vi "HWAsyncLoop.vi"(5 "HAL":refnum<queue>, 6 "Index":u32, 7 "HWAsync":refnum<queue>, 8 "error in":errorcluster, 10 "Async ACQ Notifier in":refnum<notifier>) -> (0 "error out":errorcluster)   [LabVIEW 2014, in "HWAsyncLoop.lvlib"]
uses:
  HWAsyncLoop.lvlib
  APIs/Message Queue/Message Cluster.ctl
  APIs/Data Queue/Async Acquisition Data Cluster.ctl
  DriverMasterAsync/builds/DriverMasterAsync.lvlibp/Modules/HAL/DriverMasterAsync/DriverMasterAsyncClass/DriverMasterAsync.lvclass
  Typedefs/HWAsync State.ctl
  <vilib>/Utility/error.llb/DialogType.ctl
  APIs/Message Queue/Enqueue Message (Single).vi
  <vilib>/Utility/LVLibp/NI_PackedLibraryUtility.lvlib
  APIs/Message Queue/WINFAS 2 Message Queue.lvlib
  APIs/Data Queue/WINFAS 2 Data Queue.lvlib
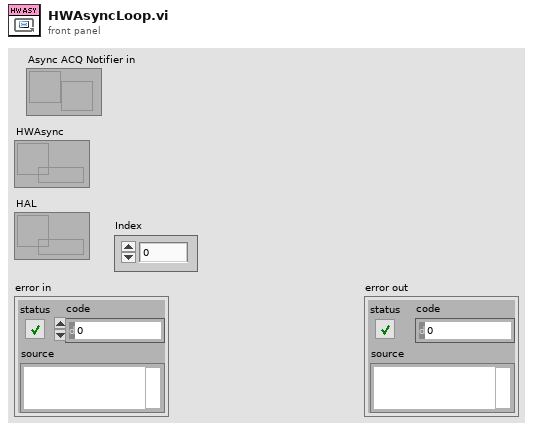
[diagram p1: front panel]
types:
  T1 = typedef "HWAsyncLoop.lvlib/HWAsync State.ctl" = enum16{"INIT", "Off", "Idle", "ACQ"}
  T2 = typedef "DialogType.ctl" = u16
  T3 = typedef "DriverMasterAsync.lvlibp/WINFAS 2 Data Queue.lvlib/Async Acquisition Data Cluster.ctl" = cluster{"Data":sgl[]}
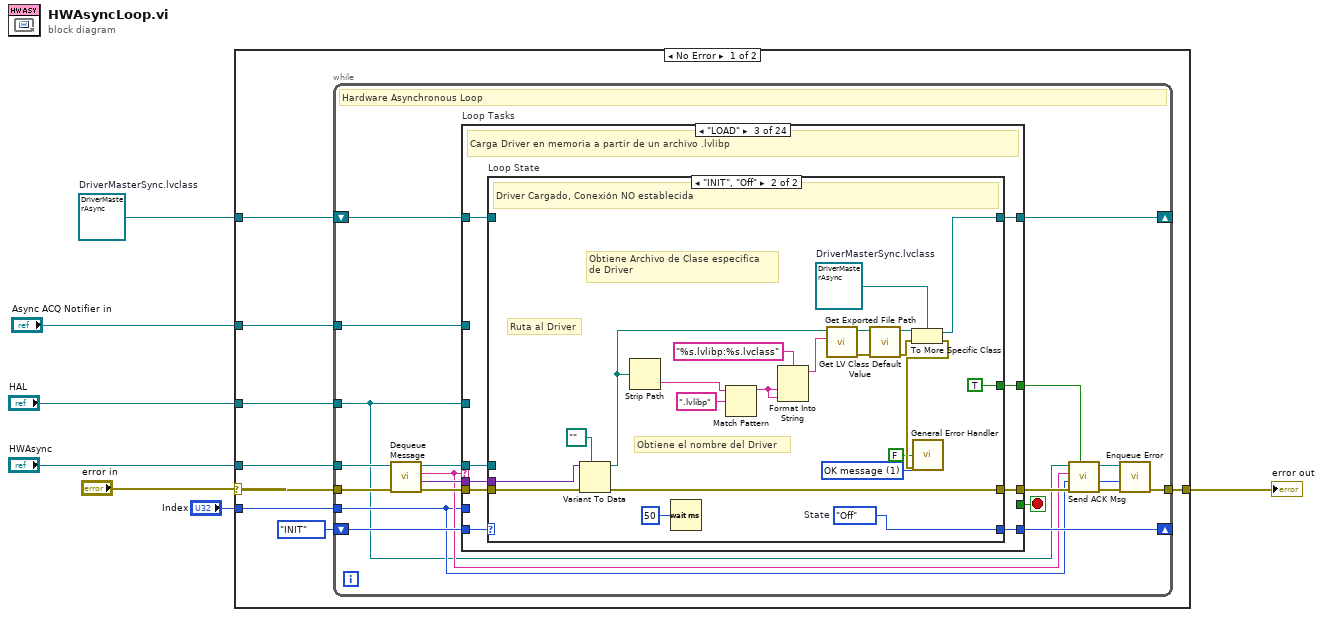
[diagram p0: block diagram]
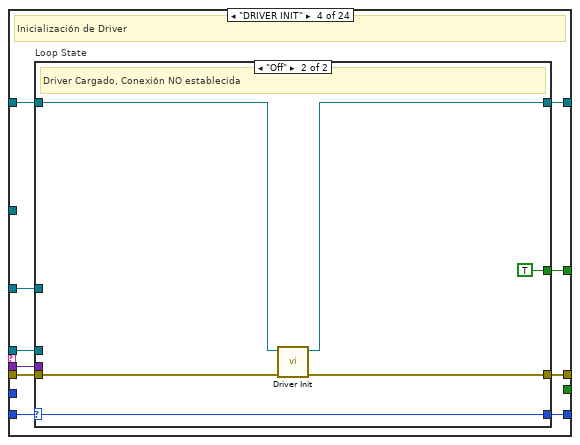
[diagram p5: hidden frame]
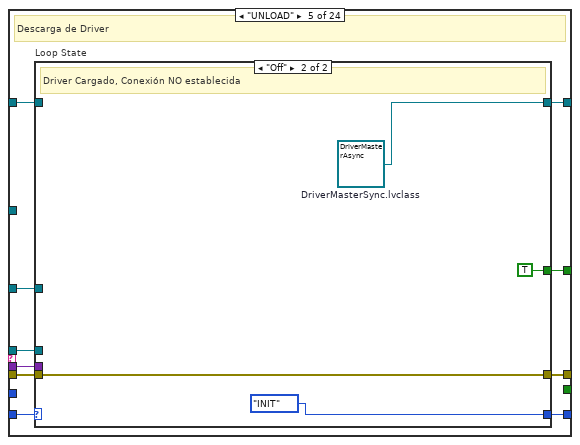
[diagram p7: hidden frame]
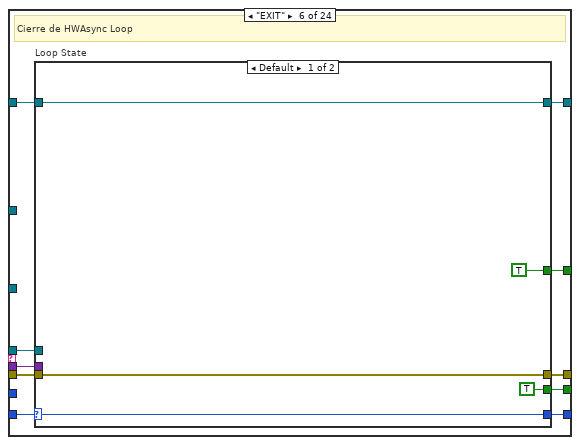
[diagram p9: hidden frame]
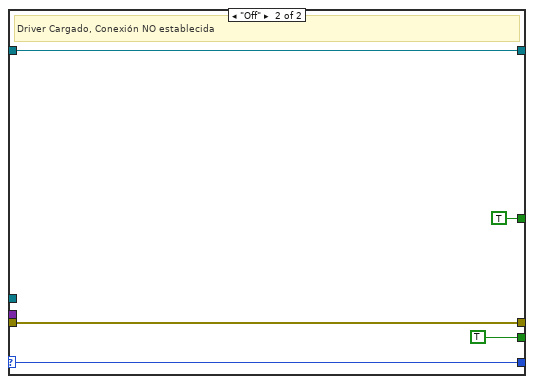
[diagram p10: hidden frame]
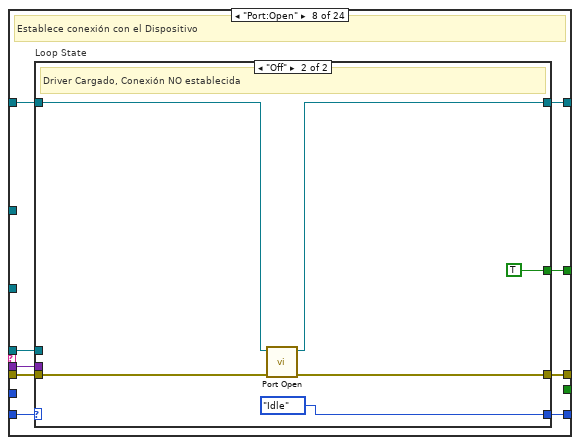
[diagram p12: hidden frame]
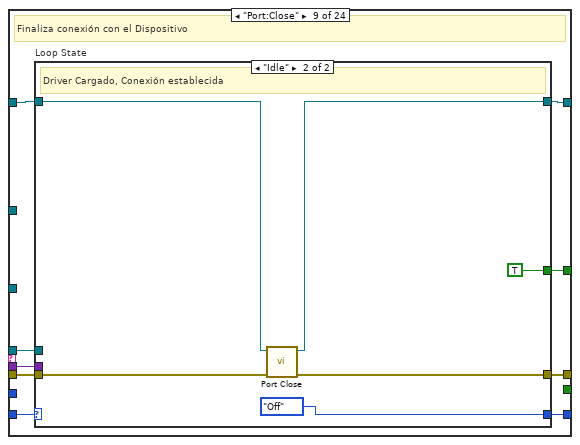
[diagram p14: hidden frame]
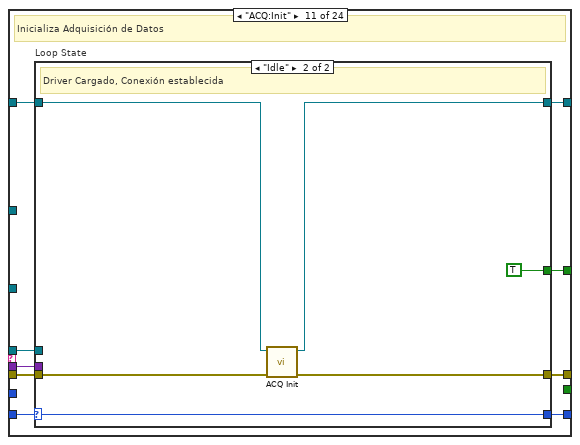
[diagram p17: hidden frame]
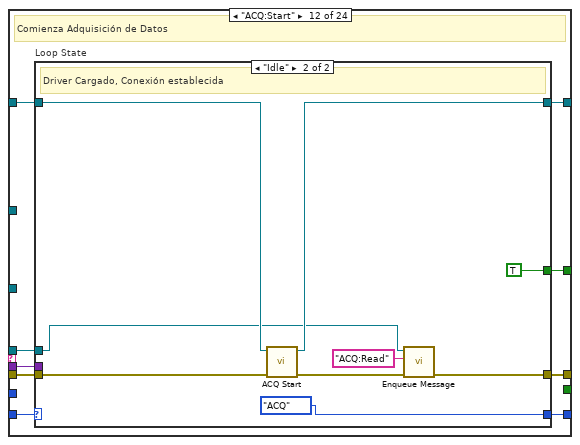
[diagram p19: hidden frame]
diagram:
  w3 = refnum<class "DriverMasterAsync.lvclass"> refnum  # DriverMasterSync.lvclass
  n1 = case shown="No Error" "error in" {
    selector: "error in" -> [w15 w435]
    tunnel: [w11 w435] -> w6
    tunnel: "HWAsync" -> [w14 _]
    tunnel: "HAL" -> [w12 _]
    tunnel: w3 -> [w10 _]
    tunnel: "Index" -> [w9 _]
    tunnel: "Async ACQ Notifier in" -> [w8 _]
    frame No Error {
      n2 = while {
        tunnel: w15 -> [w35]
        tunnel: w14 -> [w21]
        shift-right: [w30] -> _
        shift-left: HWAsync_State."INIT" ("State") -> [w29]
        tunnel: w12 -> [w17]
        tunnel: [w26] -> w11
        shift-right: [w32] -> _
        shift-left: w10 -> [w27]
        tunnel: w9 -> [w19]
        tunnel: w8 -> [w16]
        stop <- w34 stop-if-true
        # "Hardware Asynchronous Loop"
        n3 = call "Dequeue Message.vi"("error in (no error)"=w35, "Message Queue"=w21) -> ("error out"=w33:errorcluster, "Message Data"=w31:variant, "Message"=w20:string, "dup Message Queue"=w28:refnum<queue>)  [unwired: 6 in]
        n4 = case "Loop Tasks" shown="\"LOAD\"" w20 {
          tunnel: w28 -> [_ _ w46 w81 w100 w117 _ w139 w157 _ w178 w196 w219 w250 w269 _ w295 w313 w331 _ w353 w375 w396 w421]
          tunnel: w17 -> [_ _ _ w77 w96 _ _ _ _ _ _ _ w215 _ _ _ _ _ _ _ w349 w371 w392 w417]
          tunnel: [_ _ _ _ _ w113 _ _ _ _ _ _ _ _ _ _ _ _ _ _ _ _ _ _] -> w34
          tunnel: w33 -> [w38 w41 w49 w84 w103 w120 w134 w142 w160 w173 w181 w199 w222 w253 w272 w290 w298 w316 w334 w347 w356 w378 w399 w424]
          tunnel: [w38 w41 w47 w82 w101 w118 w134 w140 w158 w173 w179 w197 w220 w251 w270 w290 w296 w314 w332 w347 w354 w376 w397 w422] -> w22
          tunnel: w27 -> [w37 w40 w44 w79 w98 w115 w133 w137 w155 w172 w176 w194 w217 w248 w267 w289 w293 w311 w329 w346 w351 w373 w394 w419]
          tunnel: [w37 w40 w50 w85 w104 w121 w133 w143 w161 w172 w182 w200 w223 w254 w273 w289 w299 w317 w335 w346 w357 w379 w400 w425] -> w32
          tunnel: w31 -> [_ _ w48 w83 w102 w119 _ w141 w159 _ w180 w198 w221 w252 w271 _ w297 w315 w333 _ w355 w377 w398 w423]
          tunnel: [w36 w39 w43 w78 w97 w114 w132 w136 w154 w171 w175 w193 w216 w247 w266 w288 w292 w310 w328 w345 w350 w372 w393 w418] -> w30
          tunnel: w29 -> [w36 w39 w45 w80 w99 w116 w132 w138 w156 w171 w177 w195 w218 w249 w268 w288 w294 w312 w330 w345 w352 w374 w395 w420]
          tunnel: w19 -> [_ _ _ _ _ _ _ _ _ _ _ _ w214 _ _ _ _ _ _ _ _ _ w390 _]
          tunnel: [_ _ w42 w76 w95 w112 _ w135 w153 _ w174 w192 _ w246 w265 _ w291 w309 w327 _ w348 w370 w391 w416] -> w18
          tunnel: w16 -> [_ _ _ _ _ _ _ _ _ _ _ _ w213 _ w264 _ _ _ _ _ _ _ _ _]
          frame "----LOOP----" {
          }
          frame Default {
          }
          frame "LOAD" {
            # "Carga Driver en memoria a partir de un archivo .lvlibp"
            n5 = case "Loop State" shown="\"INIT\", \"Off\"" w45 {
              selector: w45 -> [w51 _]
              tunnel: [w53 w70] -> w50
              tunnel: w49 -> [w52 w69]
              tunnel: w48 -> [_ w68]
              tunnel: [w52 w59] -> w47
              tunnel: w46 -> [_ _]
              tunnel: w44 -> [w53 _]
              tunnel: [w51 w61] -> w43
              tunnel: [_ TRUE] -> w42
              frame Default {
              }
              frame "INIT", "Off" {
                w54 = T2 1 items=["no dialog", "OK message", "continue or stop message", "OK message + warnings", "continue/stop + warnings"] ("type of dialog (OK msg:1)")
                w61 = HWAsync_State."Off"  # State
                w71 = refnum<class "DriverMasterAsync.lvclass"> refnum  # DriverMasterSync.lvclass
                # "Ruta al Driver"
                # "Obtiene el nombre del Driver"
                # "Obtiene Archivo de Clase especifica\nde Driver"
                # "Driver Cargado, Conexión NO establecida"
                n6 = Variant To Data(error in=w69, type=path "", Variant=w68) -> (data=w64:path, error out=w59:errorcluster)
                n7 = Strip Path(path=w64) -> (name=w65:string)  [unwired: 1 out]
                n8 = Wait (ms)(milliseconds to wait=u32 50) -> ()  [unwired: 1 out]
                n9 = Match Pattern(string=w65, regular expression=".lvlibp") -> (before substring=w63:string)  [unwired: 1 in, 3 out]
                n10 = Format Into String(format string="%s.lvlibp:%s.lvclass", w63, w63) -> (resulting string=w74:string)  [unwired: 2 in, 1 out]
                n11 = call <vilib>:"Get Exported File Path.vi"("qualified name"=w74, "packed library path"=w64) -> ("error out"=w58:errorcluster, "path"=w75:path)  [unwired: 8 in]
                n12 = call <vilib>:"Get LV Class Default Value.vi"("error in (no error)"=w58, "class path"=w75) -> ("error out"=w57:errorcluster, "object"=w73:refnum<class>)  [unwired: 8 in]
                n13 = To More Specific Class(target class=w71, reference=w73, error in=w57) -> (specific class reference=w70:refnum<class "DriverMasterAsync.lvclass">, error out=w56:errorcluster)
                n14 = call <vilib>:"General Error Handler.vi"("search ni.com link visible?(T)"=FALSE, "type of dialog (OK msg:1)"=w54, "error in (no error)"=w56) -> ()  [unwired: 8 in, 5 out]
              }
            }
          }
          frame "DRIVER INIT" {
            # "Inicialización de Driver"
            n15 = case "Loop State" shown="\"Off\"" w80 {
              selector: w80 -> [w86 w94]
              tunnel: [w88 w91] -> w85
              tunnel: w84 -> [w87 w93]
              tunnel: w83 -> [_ _]
              tunnel: [w87 w89] -> w82
              tunnel: w81 -> [_ _]
              tunnel: w79 -> [w88 w92]
              tunnel: [w86 w94] -> w78
              tunnel: w77 -> [_ _]
              tunnel: [_ TRUE] -> w76
              frame Default {
              }
              frame "Off" {
                # "Driver Cargado, Conexión NO establecida"
                n16 = call-dynamic "Driver Init.vi"("error in (no error)"=w93, "DriverMasterAsync in"=w92) -> ("error out"=w89:errorcluster, "DriverMasterAsync out"=w91:refnum<class "DriverMasterAsync.lvclass">)  [unwired: 8 in]
              }
            }
          }
          frame "UNLOAD" {
            # "Descarga de Driver"
            n17 = case "Loop State" shown="\"Off\"" w99 {
              selector: w99 -> [w105 _]
              tunnel: [w107 w110] -> w104
              tunnel: w103 -> [w106 w109]
              tunnel: w102 -> [_ _]
              tunnel: [w106 w109] -> w101
              tunnel: w100 -> [_ _]
              tunnel: w98 -> [w107 _]
              tunnel: [w105 HWAsync_State."INIT" ("State")] -> w97
              tunnel: w96 -> [_ _]
              tunnel: [_ TRUE] -> w95
              frame Default {
              }
              frame "Off" {
                w110 = refnum<class "DriverMasterAsync.lvclass"> refnum  # DriverMasterSync.lvclass
                # "Driver Cargado, Conexión NO establecida"
              }
            }
          }
          frame "EXIT" {
            # "Cierre de HWAsync Loop"
            n18 = case "Loop State" shown="Default" w116 {
              selector: w116 -> [w124 w128]
              tunnel: [w126 w130] -> w121
              tunnel: w120 -> [w125 w129]
              tunnel: w119 -> [_ _]
              tunnel: [w125 w129] -> w118
              tunnel: w117 -> [_ _]
              tunnel: w115 -> [w126 w130]
              tunnel: [w124 w128] -> w114
              tunnel: [TRUE TRUE] -> w113
              tunnel: [TRUE TRUE] -> w112
              frame Default {
              }
              frame "Off" {
                # "Driver Cargado, Conexión NO establecida"
              }
            }
          }
          frame "----PORT----" {
          }
          frame "Port:Open" {
            # "Establece conexión con el Dispositivo"
            n19 = case "Loop State" shown="\"Off\"" w138 {
              selector: w138 -> [w144 _]
              tunnel: [w146 w149] -> w143
              tunnel: w142 -> [w145 w152]
              tunnel: w141 -> [_ _]
              tunnel: [w145 w151] -> w140
              tunnel: w139 -> [_ _]
              tunnel: w137 -> [w146 w150]
              tunnel: [w144 HWAsync_State."Idle" ("State")] -> w136
              tunnel: [_ TRUE] -> w135
              frame Default {
              }
              frame "Off" {
                # "Driver Cargado, Conexión NO establecida"
                n20 = call-dynamic "Port Open.vi"("error in (no error)"=w152, "DriverMasterAsync in"=w150) -> ("error out"=w151:errorcluster, "DriverMasterAsync out"=w149:refnum<class "DriverMasterAsync.lvclass">)  [unwired: 8 in]
              }
            }
          }
          frame "Port:Close" {
            # "Finaliza conexión con el Dispositivo"
            n21 = case "Loop State" shown="\"Idle\"" w156 {
              selector: w156 -> [w162 _]
              tunnel: [w164 w167] -> w161
              tunnel: w160 -> [w163 w170]
              tunnel: w159 -> [_ _]
              tunnel: [w163 w169] -> w158
              tunnel: w157 -> [_ _]
              tunnel: w155 -> [w164 w168]
              tunnel: [w162 HWAsync_State."Off" ("State")] -> w154
              tunnel: [_ TRUE] -> w153
              frame Default {
              }
              frame "Idle" {
                # "Driver Cargado, Conexión establecida"
                n22 = call-dynamic "Port Close.vi"("error in (no error)"=w170, "DriverMasterAsync in"=w168) -> ("error out"=w169:errorcluster, "DriverMasterAsync out"=w167:refnum<class "DriverMasterAsync.lvclass">)  [unwired: 8 in]
              }
            }
          }
          frame "----ACQ----" {
          }
          frame "ACQ:Init" {
            # "Inicializa Adquisición de Datos"
            n23 = case "Loop State" shown="\"Idle\"" w177 {
              selector: w177 -> [w183 w186]
              tunnel: [w185 w189] -> w182
              tunnel: w181 -> [w184 w191]
              tunnel: w180 -> [_ _]
              tunnel: [w184 w187] -> w179
              tunnel: w178 -> [_ _]
              tunnel: w176 -> [w185 w190]
              tunnel: [w183 w186] -> w175
              tunnel: [_ TRUE] -> w174
              frame Default {
              }
              frame "Idle" {
                # "Driver Cargado, Conexión establecida"
                n24 = call-dynamic "ACQ Init.vi"("error in (no error)"=w191, "DriverMasterAsync in"=w190) -> ("error out"=w187:errorcluster, "DriverMasterAsync out"=w189:refnum<class "DriverMasterAsync.lvclass">)  [unwired: 8 in]
              }
            }
          }
          frame "ACQ:Start" {
            # "Comienza Adquisición de Datos"
            n25 = case "Loop State" shown="\"Idle\"" w195 {
              selector: w195 -> [w201 _]
              tunnel: [w203 w210] -> w200
              tunnel: w199 -> [w202 w212]
              tunnel: w198 -> [_ _]
              tunnel: [w202 w206] -> w197
              tunnel: w196 -> [_ w205]
              tunnel: w194 -> [w203 w211]
              tunnel: [w201 HWAsync_State."ACQ" ("State")] -> w193
              tunnel: [_ TRUE] -> w192
              frame Default {
              }
              frame "Idle" {
                # "Driver Cargado, Conexión establecida"
                n26 = call-dynamic "ACQ Start.vi"("error in (no error)"=w212, "DriverMasterAsync in"=w211) -> ("error out"=w207:errorcluster, "DriverMasterAsync out"=w210:refnum<class "DriverMasterAsync.lvclass">)  [unwired: 8 in]
                n27 = call-poly "Enqueue Message.vi"("error in (no error)"=w207, "Message"="ACQ:Read", "Message Queue"=w205) -> ("error out"=w206:errorcluster)  [unwired: 7 in, 1 out]
              }
            }
          }
          frame "ACQ:Read" {
            # "Adquiere Datos"
            n28 = case "Loop State" shown="\"ACQ\"" w218 {
              selector: w218 -> [w224 w239]
              tunnel: [w226 w236] -> w223
              tunnel: w222 -> [w225 w241]
              tunnel: w221 -> [_ _]
              tunnel: [w225 w227] -> w220
              tunnel: w219 -> [_ w234]
              tunnel: w217 -> [w226 w240]
              tunnel: [w224 w239] -> w216
              tunnel: w215 -> [_ _]
              tunnel: w214 -> [_ _]
              tunnel: w213 -> [_ w230]
              frame Default {
              }
              frame "ACQ" {
                # "Adquiriendo Datos"
                n29 = for {
                  N: 100 -> [_]
                  tunnel: w240 -> [w244]
                  tunnel: [w243] -> w237
                  tunnel: w241 -> [w245]
                  tunnel: [w242] -> w238
                  stop <- w242 continue-if-true
                  n30 = call-dynamic "ACQ Read.vi"("error in (no error)"=w245, "DriverMasterAsync in"=w244) -> ("error out"=w242:errorcluster, "DriverMasterAsync out"=w243:refnum<class "DriverMasterAsync.lvclass">)  [unwired: 8 in]
                }
                n31 = call "Read ACQ Data.vi"("error in (no error)"=w238, "DriverMasterAsync in"=w237) -> ("error out"=w232:errorcluster, "ACQ Data"=w231:T3, "DriverMasterAsync out"=w236:refnum<class "DriverMasterAsync.lvclass">)  [unwired: 7 in]
                n32 = call "Send Async ACQ Notification.vi"("error in (no error)"=w232, "Async ACQ"=w231, "Async ACQ Notifier in"=w230) -> ("error out"=w229:errorcluster)  [unwired: 7 in, 1 out]
                n33 = call-poly "Enqueue Message.vi"("error in (no error)"=w232, "Message"="ACQ:Read", "Message Queue"=w234) -> ("error out"=w228:errorcluster)  [unwired: 7 in, 1 out]
                n34 = Merge Errors(w229, w228) -> (w227:errorcluster)
              }
            }
          }
          frame "ACQ:Stop" {
            # "Detiene Adquisición de Datos"
            n35 = case "Loop State" shown="\"ACQ\"" w249 {
              selector: w249 -> [w255 _]
              tunnel: [w257 w260] -> w254
              tunnel: w253 -> [w256 w263]
              tunnel: w252 -> [_ _]
              tunnel: [w256 w262] -> w251
              tunnel: w250 -> [_ _]
              tunnel: w248 -> [w257 w261]
              tunnel: [w255 HWAsync_State."Idle" ("State")] -> w247
              tunnel: [_ TRUE] -> w246
              frame Default {
              }
              frame "ACQ" {
                # "Adquiriendo Datos"
                n36 = call-dynamic "ACQ Stop.vi"("error in (no error)"=w263, "DriverMasterAsync in"=w261) -> ("error out"=w262:errorcluster, "DriverMasterAsync out"=w260:refnum<class "DriverMasterAsync.lvclass">)  [unwired: 8 in]
              }
            }
          }
          frame "Auto-Cycle" {
            # "Comienza Adquisición de Datos Automatica"
            n37 = case "Loop State" shown="\"Idle\"" w268 {
              selector: w268 -> [w274 w284]
              tunnel: [w276 w281] -> w273
              tunnel: w272 -> [w275 w287]
              tunnel: w271 -> [_ _]
              tunnel: [w275 w279] -> w270
              tunnel: w269 -> [_ _]
              tunnel: w267 -> [w276 w286]
              tunnel: [w274 w284] -> w266
              tunnel: [_ TRUE] -> w265
              tunnel: w264 -> [_ w277]
              frame Default {
              }
              frame "Idle" {
                # "Driver Cargado, Conexión establecida"
                n38 = call-dynamic "Auto-Cycle.vi"("error in (no error)"=w287, "DriverMasterAsync in"=w286) -> ("error out"=w283:errorcluster, "DriverMasterAsync out"=w282:refnum<class "DriverMasterAsync.lvclass">)  [unwired: 8 in]
                n39 = call "Read ACQ Data.vi"("error in (no error)"=w283, "DriverMasterAsync in"=w282) -> ("error out"=w280:errorcluster, "ACQ Data"=w278:T3, "DriverMasterAsync out"=w281:refnum<class "DriverMasterAsync.lvclass">)  [unwired: 7 in]
                n40 = call "Send Async ACQ Notification.vi"("error in (no error)"=w280, "Async ACQ"=w278, "Async ACQ Notifier in"=w277) -> ("error out"=w279:errorcluster)  [unwired: 7 in, 1 out]
              }
            }
          }
          frame "----ACTION----" {
          }
          frame "Action:Init" {
            # "Inicializa Parametros de Funciones"
            n41 = case "Loop State" shown="\"Idle\"" w294 {
              selector: w294 -> [w300 w304]
              tunnel: [w302 w306] -> w299
              tunnel: w298 -> [w301 w308]
              tunnel: w297 -> [_ _]
              tunnel: [w301 w303] -> w296
              tunnel: w295 -> [_ _]
              tunnel: w293 -> [w302 w307]
              tunnel: [w300 w304] -> w292
              tunnel: [_ TRUE] -> w291
              frame Default {
              }
              frame "Idle" {
                # "Driver Cargado, Conexión establecida"
                n42 = call-dynamic "Action Init.vi"("error in (no error)"=w308, "DriverMasterAsync in"=w307) -> ("error out"=w303:errorcluster, "DriverMasterAsync out"=w306:refnum<class "DriverMasterAsync.lvclass">)  [unwired: 8 in]
              }
            }
          }
          frame "Action:1" {
            # "Realiza Función 1"
            n43 = case "Loop State" shown="\"Idle\"" w312 {
              selector: w312 -> [w318 w322]
              tunnel: [w320 w324] -> w317
              tunnel: w316 -> [w319 w326]
              tunnel: w315 -> [_ _]
              tunnel: [w319 w321] -> w314
              tunnel: w313 -> [_ _]
              tunnel: w311 -> [w320 w325]
              tunnel: [w318 w322] -> w310
              tunnel: [_ TRUE] -> w309
              frame Default {
              }
              frame "Idle" {
                # "Driver Cargado, Conexión establecida"
                n44 = call-dynamic "Action 1.vi"("error in (no error)"=w326, "DriverMasterAsync in"=w325) -> ("error out"=w321:errorcluster, "DriverMasterAsync out"=w324:refnum<class "DriverMasterAsync.lvclass">)  [unwired: 8 in]
              }
            }
          }
          frame "Action:2" {
            # "Realiza Función 2"
            n45 = case "Loop State" shown="\"Idle\"" w330 {
              selector: w330 -> [w336 w340]
              tunnel: [w338 w342] -> w335
              tunnel: w334 -> [w337 w344]
              tunnel: w333 -> [_ _]
              tunnel: [w337 w339] -> w332
              tunnel: w331 -> [_ _]
              tunnel: w329 -> [w338 w343]
              tunnel: [w336 w340] -> w328
              tunnel: [_ TRUE] -> w327
              frame Default {
              }
              frame "Idle" {
                # "Driver Cargado, Conexión establecida"
                n46 = call-dynamic "Action 2.vi"("error in (no error)"=w344, "DriverMasterAsync in"=w343) -> ("error out"=w339:errorcluster, "DriverMasterAsync out"=w342:refnum<class "DriverMasterAsync.lvclass">)  [unwired: 8 in]
              }
            }
          }
          frame "----UTILITY----" {
          }
          frame "Config" {
            # "Abre Panel de Configuración de Driver"
            n47 = case "Loop State" shown="\"Off\"" w352 {
              selector: w352 -> [w358 w369]
              tunnel: [w360 w362] -> w357
              tunnel: w356 -> [w359 w365]
              tunnel: w355 -> [_ _]
              tunnel: [w359 w368] -> w354
              tunnel: w353 -> [_ _]
              tunnel: w351 -> [w360 w363]
              tunnel: [w358 w369] -> w350
              tunnel: w349 -> [_ w367]
              tunnel: [_ TRUE] -> w348
              frame Default {
              }
              frame "Off" {
                # "HAL Config Data"
                # "Driver Cargado, Conexión NO establecida"
                n48 = call-dynamic "Config.vi"("error in (no error)"=w365, "DriverMasterAsync in"=w363) -> ("error out"=w364:errorcluster, "DriverMasterAsync out"=w362:refnum<class "DriverMasterAsync.lvclass">)  [unwired: 8 in]
                n49 = call-poly "Enqueue Message.vi"("error in (no error)"=w364, "Message"="Update Driver Config", "Message Queue"=w367) -> ("error out"=w368:errorcluster)  [unwired: 7 in, 1 out]
              }
            }
          }
          frame "Config:Set" {
            # "Setea Configuración desde afuera"
            n50 = case "Loop State" shown="\"Off\"" w374 {
              selector: w374 -> [w380 w389]
              tunnel: [w382 w386] -> w379
              tunnel: w378 -> [w381 w388]
              tunnel: w377 -> [_ w384]
              tunnel: [w381 w383] -> w376
              tunnel: w375 -> [_ _]
              tunnel: w373 -> [w382 w387]
              tunnel: [w380 w389] -> w372
              tunnel: w371 -> [_ _]
              tunnel: [_ TRUE] -> w370
              frame Default {
              }
              frame "Off" {
                # "Driver Cargado, Conexión NO establecida"
                n51 = call-dynamic "Set Config.vi"("error in (no error)"=w388, "Config Data"=w384, "DriverMasterAsync in"=w387) -> ("error out"=w383:errorcluster, "DriverMasterAsync out"=w386:refnum<class "DriverMasterAsync.lvclass">)  [unwired: 7 in]
              }
            }
          }
          frame "Config:Get" {
            # "Envía Configuración hacia afuera"
            n52 = case "Loop State" shown="\"Off\"" w395 {
              selector: w395 -> [w401 w415]
              tunnel: [w403 w412] -> w400
              tunnel: w399 -> [w402 w414]
              tunnel: w398 -> [_ _]
              tunnel: [w402 w408] -> w397
              tunnel: w396 -> [_ _]
              tunnel: w394 -> [w403 w413]
              tunnel: [w401 w415] -> w393
              tunnel: w392 -> [_ w407]
              tunnel: [_ TRUE] -> w391
              tunnel: w390 -> [_ w406]
              frame Default {
              }
              frame "Off" {
                # "Driver Cargado, Conexión NO establecida"
                n53 = call-dynamic "Get Config.vi"("error in (no error)"=w414, "DriverMasterAsync in"=w413) -> ("error out"=w409:errorcluster, "Config Data"=w404:variant, "DriverMasterAsync out"=w412:refnum<class "DriverMasterAsync.lvclass">)  [unwired: 7 in]
                n54 = Format Into String(format string="CONFIG:HWAsync:%d" ("Message"), w406) -> (resulting string=w410:string)  [unwired: 2 in, 1 out]
                n55 = call-poly "Enqueue Message.vi"("error in (no error)"=w409, "Message Data"=w404, "Message"=w410, "Message Queue"=w407) -> ("error out"=w408:errorcluster)  [unwired: 6 in, 1 out]
              }
            }
          }
          frame "Auto-Zero" {
            # "Realiza Cerado del sensor"
            n56 = case "Loop State" shown="\"Idle\"" w420 {
              selector: w420 -> [w426 w434]
              tunnel: [w428 w431] -> w425
              tunnel: w424 -> [w427 w433]
              tunnel: w423 -> [_ _]
              tunnel: [w427 w429] -> w422
              tunnel: w421 -> [_ _]
              tunnel: w419 -> [w428 w432]
              tunnel: [w426 w434] -> w418
              tunnel: w417 -> [_ _]
              tunnel: [_ TRUE] -> w416
              frame Default {
              }
              frame "Idle" {
                # "HAL Config Data"
                # "Driver Cargado, Conexión establecida"
                n57 = call-dynamic "Auto-Zero.vi"("error in (no error)"=w433, "DriverMasterAsync in"=w432) -> ("error out"=w429:errorcluster, "DriverMasterAsync out"=w431:refnum<class "DriverMasterAsync.lvclass">)  [unwired: 8 in]
              }
            }
          }
        }
        n58 = call "Send ACK Msg.vi"("Enable?"=w18, "error in (no error)"=w22, "Index"=w19, "Message"=w20, "HAL  in"=w17) -> ("error out"=w24:errorcluster, "dup Index"=w23:u32, "HAL  out"=w25:refnum<queue>)  [unwired: 4 in]
        n59 = call "Enqueue Error.vi"("Error In"=w24, "Index"=w23, "HAL Message Queue"=w25) -> ("dup Error Out"=w26:errorcluster)  [unwired: 8 in]
      }
    }
    frame Error {
    }
  }
  "error out" <- w6
